vi "All Services.vi"(8 "error in (no error)":errorcluster, 11 "Service Container in":refnum<class "Service Container.lvclass">) -> (0 "error out":errorcluster, 2 "Services":refnum<class "Service.lvclass">[](array[class]), 3 "Service Container out":refnum<class "Service Container.lvclass">)   [LabVIEW 2020, in "Vecto.lvlib" / "Service Container.lvclass"]
uses:
  Service Container.lvclass
  Service/Service.lvclass
  Service Container.lvclass/Service Container.ctl
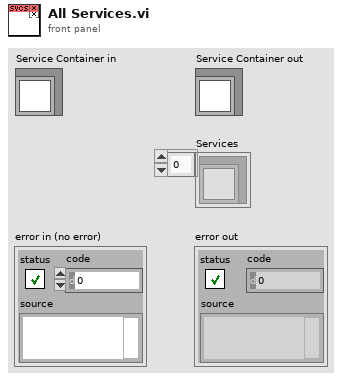
[diagram p1: front panel]
types:
  T1 = typedef "Vecto.lvlib/Service Container.lvclass/Services.ctl" = map{string, map{string, refnum<class "Service.lvclass">}}
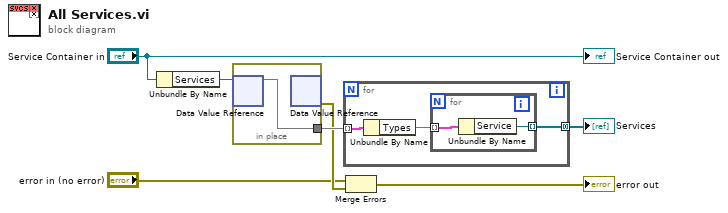
[diagram p0: block diagram]
diagram:
  n1 = Unbundle By Name("Service Container in") -> ("Services"=w7:refnum<data-value>)
  n2 = in-place {
    in-place-border: [w8] -> w6
    n3 = in-place-dvr #1(w7) -> (w8:T1)  [unwired: 1 out]
    n4 = in-place-dvr #1() -> (w4:errorcluster)  [unwired: 1 in, 1 out]
  }
  n5 = for {
    tunnel: [w10] -> w5 mode=concatenating
    tunnel: w6 -> [w9] mode=indexing
    n6 = Unbundle By Name(w9) -> ("Types"=w11:map{string, refnum<class "Service.lvclass">})
    n7 = for {
      tunnel: w11 -> [w12] mode=indexing
      tunnel: [w13] -> w10 mode=indexing
      n8 = Unbundle By Name(w12) -> ("Service"=w13:refnum<class "Service.lvclass">)
    }
  }
  "Services" <- w5
  n9 = Merge Errors("error in (no error)", w4) -> (→"error out":errorcluster)
  "Service Container out" <- "Service Container in"
